vi "例4.17-1 利用局部变量实现无else的if 语句.vi"() -> ()   [LabVIEW 2017]
panel:
  out "y":dbl
  out "y0":dbl
  in  "x":dbl
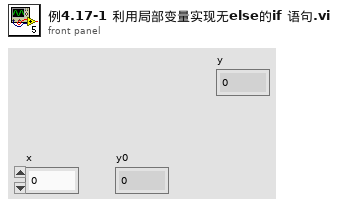
[diagram p1: front panel]
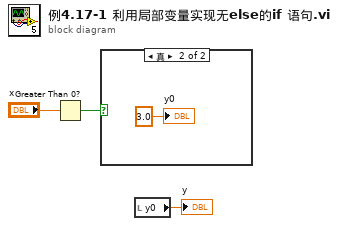
[diagram p0: block diagram]
diagram:
  n1 = Greater Than 0?(x="x") -> (x > 0?=w3:bool)
  n2 = case shown="真" w3 {
    frame False {
    }
    frame True {
      "y0" <- 3.0 ("y")
    }
  }
  n3 = local read "y0"() -> (→"y":dbl)
